vi "Get PID and Name.vi"(8 "error in (no error)":errorcluster) -> (0 "error out":errorcluster, 1 "Name":string, 2 "PID":u32)   [LabVIEW 2021, in "CIF Engine Launch.lvlib"]
uses:
  CIF Engine Launch.lvlib
  kernel32.dll
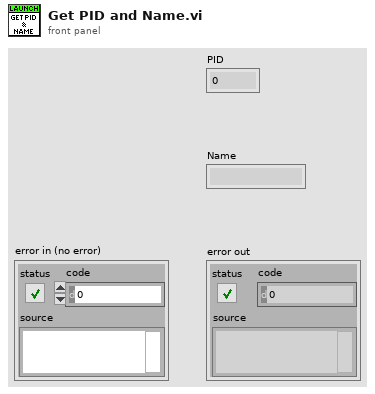
[diagram p1: front panel]
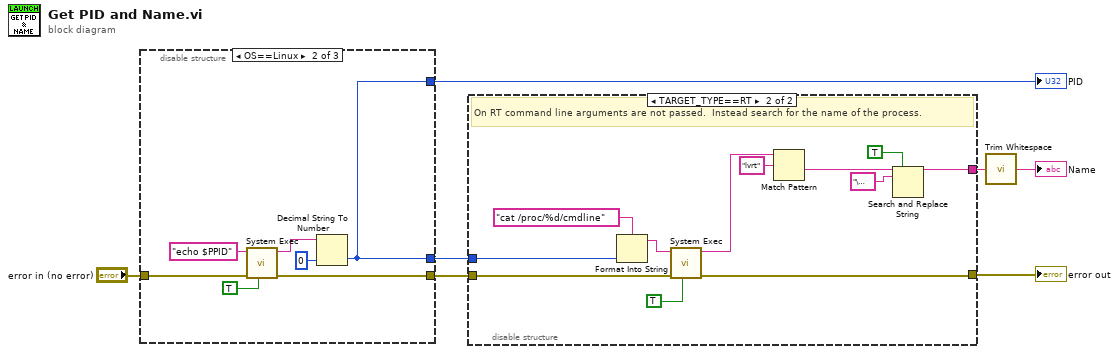
[diagram p0: block diagram]
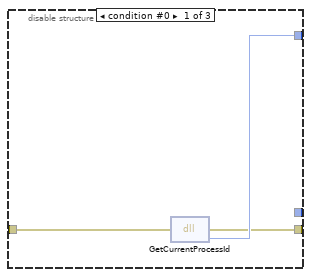
[diagram p2: hidden frame]
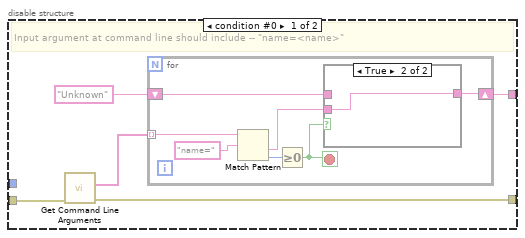
[diagram p4: hidden frame]
diagram:
  n1 = disable-structure shown="OS==Linux" {
    disable-tunnel: [w10 w11 _] -> w4
    disable-tunnel: [w9 w17 w18] -> w7
    disable-tunnel: "error in (no error)" -> [w8 w12 w18]
    disable-tunnel: [_ w11 _] -> w1
    frame condition #0 {
      n2 = dll-call lib="kernel32.dll" fn="GetCurrentProcessId"(error in=w8) -> (error out=w9:errorcluster, "return type"=w10:u32)  [unwired: 2 in, 1 out]
    }
    frame condition #1 (active) {
      n3 = call <vilib>:"System Exec.vi"("run minimized? (F)"=TRUE, "error in (no error)"=w12, "command line"="echo $PPID") -> ("error out"=w17:errorcluster, "standard output"=w13:string)  [unwired: 5 in, 2 out]
      n4 = Decimal String To Number(string=w13, default (0L)=u32 0 ("default (0 I32)")) -> (number=w11:u32)  [unwired: 1 in, 1 out]
    }
    frame condition #2 {
    }
  }
  "PID" <- w4
  n5 = disable-structure shown="TARGET_TYPE==RT" {
    disable-tunnel: [w21 w33] -> w3
    disable-tunnel: w7 -> [w20 w43]
    disable-tunnel: [w19 w42] -> w5
    disable-tunnel: w1 -> [_ w38]
    frame condition #0 {
      # "Input argument at command line should include -- \"name=<name>\""
      n6 = call <vilib>:"Get Command Line Arguments.vi"("error in (no error)"=w20) -> ("error out"=w19:errorcluster, "arguments"=w23:string[])  [unwired: 8 in, 1 out]
      n7 = for {
        tunnel: w23 -> [w30] mode=indexing
        shift-right: [w24] -> w21
        shift-left: "Unknown" -> [w27]
        stop <- w26 stop-if-true
        n8 = Match Pattern(string=w30, regular expression="name=") -> (after substring=w25:string, offset past match=w28:i32)  [unwired: 1 in, 2 out]
        n9 = Greater Or Equal To 0?(x=w28) -> (x >= 0?=w26:bool)
        n10 = case shown="True" w26 {
          tunnel: w27 -> [w31 _]
          tunnel: w25 -> [_ w32]
          tunnel: [w31 w32] -> w24
          frame False {
          }
          frame True {
          }
        }
      }
    }
    frame condition #1 (active) {
      # "On RT command line arguments are not passed.  Instead search for the name of the process."
      n11 = Format Into String(format string="cat /proc/%d/cmdline" ("string"), w38) -> (resulting string=w39:string)  [unwired: 2 in, 1 out]
      n12 = call <vilib>:"System Exec.vi"("run minimized? (F)"=TRUE, "error in (no error)"=w43, "command line"=w39) -> ("error out"=w42:errorcluster, "standard output"=w37:string)  [unwired: 5 in, 2 out]
      n13 = Match Pattern(string=w37, regular expression="lvrt") -> (after substring=w34:string)  [unwired: 1 in, 3 out]
      n14 = Search and Replace String(replace all?=TRUE ("replace all? (F)"), input string=w34, search string="\u0000") -> (result string=w33:string)  [unwired: 5 in, 3 out]
    }
  }
  "error out" <- w5
  n15 = call <vilib>:"Trim Whitespace.vi"("string"=w3) -> ("trimmed string"=→"Name":string)  [unwired: 1 in]
